vi "projectVolume.vi"(0 "xyz order":bool, 1 "input array":u32[][][](array[numeric])) -> (2 "ZY view":u32[][](array[numeric]), 3 "XZ view":u32[][](array[numeric]), 4 "XY view":u32[][](array[numeric]))   [LabVIEW 2010]
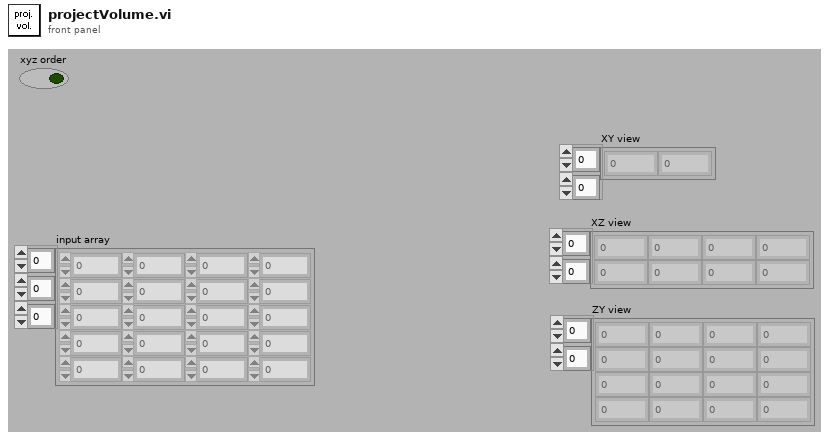
[diagram p1: front panel]
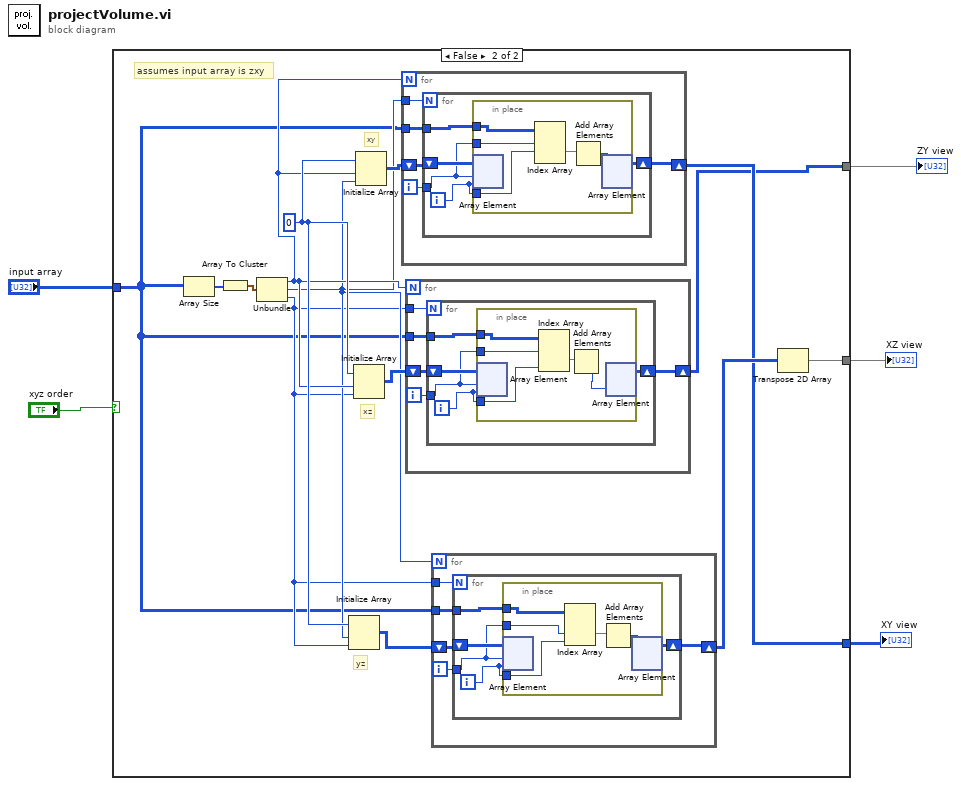
[diagram p0: block diagram]
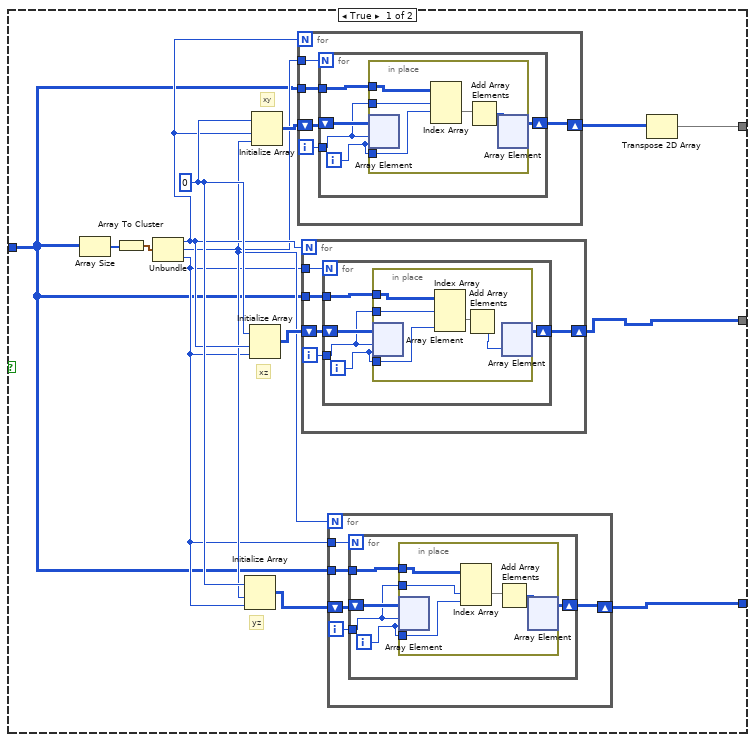
[diagram p2: hidden frame]
diagram:
  n1 = case shown="False" "xyz order" {
    tunnel: "input array" -> [w11 w70]
    tunnel: [w9 w65] -> w3
    tunnel: [w8 w67] -> w2
    tunnel: [w6 w66] -> w1
    frame True {
      w16 = u32 0
      # "yz"
      # "xz"
      # "xy"
      n2 = Array Size(array=w11) -> (size(s)=w19:i32[])
      n3 = Array To Cluster(array=w19) -> (cluster=w18:cluster{"[0]":i32, "[1]":i32, "[2]":i32})
      n4 = Unbundle(w18) -> ("[0]"=w15:i32, "[1]"=w13:i32, "[2]"=w12:i32)
      n5 = Initialize Array(w16, w13, w12) -> (w10:u32[][])
      n6 = Initialize Array(w16, w15, w12) -> (w14:u32[][])
      n7 = Initialize Array(w16, w15, w13) -> (w17:u32[][])
      n8 = for {
        N: w15 -> [_]
        tunnel: w11 -> [w53]
        tunnel: w13 -> [w52]
        shift-right: [w50] -> w7
        shift-left: w17 -> [w54]
        i -> [w51]
        n9 = for {
          N: w52 -> [_]
          tunnel: w53 -> [w58]
          tunnel: w51 -> [w57]
          shift-right: [w55] -> w50
          shift-left: w54 -> [w59]
          i -> [w56]
          n10 = in-place {
            in-place-border: w58 -> [w64]
            in-place-border: w57 -> [w63]
            in-place-border: w56 -> [w61]
            n11 = in-place-array #1(w59, w57, w56) -> ()  [unwired: 1 out]
            n12 = Index Array(array=w64, index (dim 0)=w63, index (dim 1)=w61) -> (element=w62:u32[])  [unwired: 1 in]
            n13 = Add Array Elements(numeric array=w62) -> (sum=w60:u32)
            n14 = in-place-array #1(w60) -> (w55:u32[][])  [unwired: 2 out]
          }
        }
      }
      n15 = for {
        N: w15 -> [_]
        tunnel: w11 -> [w38]
        tunnel: w12 -> [w37]
        shift-right: [w35] -> w9
        shift-left: w14 -> [w39]
        i -> [w36]
        n16 = for {
          N: w37 -> [_]
          tunnel: w38 -> [w43]
          tunnel: w36 -> [w42]
          shift-right: [w40] -> w35
          shift-left: w39 -> [w44]
          i -> [w41]
          n17 = in-place {
            in-place-border: w43 -> [w49]
            in-place-border: w42 -> [w48]
            in-place-border: w41 -> [w45]
            n18 = in-place-array #2(w44, w42, w41) -> ()  [unwired: 1 out]
            n19 = Index Array(array=w49, index (dim 0)=w48, index (dim 2)=w45) -> (element=w47:u32[])  [unwired: 1 in]
            n20 = Add Array Elements(numeric array=w47) -> (sum=w46:u32)
            n21 = in-place-array #2(w46) -> (w40:u32[][])  [unwired: 2 out]
          }
        }
      }
      n22 = for {
        N: w13 -> [_]
        tunnel: w11 -> [w23]
        tunnel: w12 -> [w22]
        shift-right: [w20] -> w8
        shift-left: w10 -> [w24]
        i -> [w21]
        n23 = for {
          N: w22 -> [_]
          tunnel: w23 -> [w28]
          tunnel: w21 -> [w27]
          shift-right: [w25] -> w20
          shift-left: w24 -> [w29]
          i -> [w26]
          n24 = in-place {
            in-place-border: w28 -> [w34]
            in-place-border: w27 -> [w30]
            in-place-border: w26 -> [w31]
            n25 = in-place-array #3(w29, w27, w26) -> ()  [unwired: 1 out]
            n26 = Index Array(array=w34, index (dim 1)=w30, index (dim 2)=w31) -> (element=w33:u32[])  [unwired: 1 in]
            n27 = Add Array Elements(numeric array=w33) -> (sum=w32:u32)
            n28 = in-place-array #3(w32) -> (w25:u32[][])  [unwired: 2 out]
          }
        }
      }
      n29 = Transpose 2D Array(2D array=w7) -> (transposed array=w6:u32[][])
    }
    frame False {
      w75 = u32 0
      # "assumes input array is zxy"
      # "yz"
      # "xz"
      # "xy"
      n30 = Array Size(array=w70) -> (size(s)=w78:i32[])
      n31 = Array To Cluster(array=w78) -> (cluster=w77:cluster{"[0]":i32, "[1]":i32, "[2]":i32})
      n32 = Unbundle(w77) -> ("[0]"=w74:i32, "[1]"=w72:i32, "[2]"=w71:i32)
      n33 = Initialize Array(w75, w72, w71) -> (w69:u32[][])
      n34 = Initialize Array(w75, w74, w71) -> (w73:u32[][])
      n35 = Initialize Array(w75, w74, w72) -> (w76:u32[][])
      n36 = for {
        N: w74 -> [_]
        tunnel: w70 -> [w112]
        tunnel: w72 -> [w111]
        shift-right: [w109] -> w67
        shift-left: w76 -> [w113]
        i -> [w110]
        n37 = for {
          N: w111 -> [_]
          tunnel: w112 -> [w117]
          tunnel: w110 -> [w116]
          shift-right: [w114] -> w109
          shift-left: w113 -> [w118]
          i -> [w115]
          n38 = in-place {
            in-place-border: w117 -> [w123]
            in-place-border: w116 -> [w122]
            in-place-border: w115 -> [w120]
            n39 = in-place-array #4(w118, w116, w115) -> ()  [unwired: 1 out]
            n40 = Index Array(array=w123, index (dim 0)=w122, index (dim 1)=w120) -> (element=w121:u32[])  [unwired: 1 in]
            n41 = Add Array Elements(numeric array=w121) -> (sum=w119:u32)
            n42 = in-place-array #4(w119) -> (w114:u32[][])  [unwired: 2 out]
          }
        }
      }
      n43 = for {
        N: w74 -> [_]
        tunnel: w70 -> [w97]
        tunnel: w71 -> [w96]
        shift-right: [w94] -> w66
        shift-left: w73 -> [w98]
        i -> [w95]
        n44 = for {
          N: w96 -> [_]
          tunnel: w97 -> [w102]
          tunnel: w95 -> [w101]
          shift-right: [w99] -> w94
          shift-left: w98 -> [w103]
          i -> [w100]
          n45 = in-place {
            in-place-border: w102 -> [w108]
            in-place-border: w101 -> [w107]
            in-place-border: w100 -> [w104]
            n46 = in-place-array #5(w103, w101, w100) -> ()  [unwired: 1 out]
            n47 = Index Array(array=w108, index (dim 0)=w107, index (dim 2)=w104) -> (element=w106:u32[])  [unwired: 1 in]
            n48 = Add Array Elements(numeric array=w106) -> (sum=w105:u32)
            n49 = in-place-array #5(w105) -> (w99:u32[][])  [unwired: 2 out]
          }
        }
      }
      n50 = for {
        N: w72 -> [_]
        tunnel: w70 -> [w82]
        tunnel: w71 -> [w81]
        shift-right: [w79] -> w68
        shift-left: w69 -> [w83]
        i -> [w80]
        n51 = for {
          N: w81 -> [_]
          tunnel: w82 -> [w87]
          tunnel: w80 -> [w86]
          shift-right: [w84] -> w79
          shift-left: w83 -> [w88]
          i -> [w85]
          n52 = in-place {
            in-place-border: w87 -> [w93]
            in-place-border: w86 -> [w89]
            in-place-border: w85 -> [w90]
            n53 = in-place-array #6(w88, w86, w85) -> ()  [unwired: 1 out]
            n54 = Index Array(array=w93, index (dim 1)=w89, index (dim 2)=w90) -> (element=w92:u32[])  [unwired: 1 in]
            n55 = Add Array Elements(numeric array=w92) -> (sum=w91:u32)
            n56 = in-place-array #6(w91) -> (w84:u32[][])  [unwired: 2 out]
          }
        }
      }
      n57 = Transpose 2D Array(2D array=w68) -> (transposed array=w65:u32[][])
    }
  }
  "ZY view" <- w1
  "XZ view" <- w3
  "XY view" <- w2
